vi "LoadWaveform.vi"() -> ()   [LabVIEW 2013]
panel:
  in  "Tab Control 2":enum32{"Main TEK", "load colored noise"}(tab)
  in  "channel 2":cluster{"output":bool}
  in  "channel 1":T1={"Modulation Waveform (1: Sine)"=200, "modulation"=FALSE, "output"=FALSE} {"Modulation Waveform (1: Sine)" items=["Sine"=1, "Square"=2, "Triangle"=3, "Ramp Up"=4, "Ramp Down"=5, "Noise"=100, "Arbitrary User1"=200, "Arbitrary User2"=201, "Arbitrary User3"=202, "Arbitrary User4"=203, "Edit Memory"=204]}
  in  "outpout mode":i32(ring) items=["Standard Waveform", "Arbitrary Waveform"]
  in  "configuration main":bool
  in  "amplitude (1)":dbl=1.0
  in  "dc offset (0.00)":dbl
  in  "frequency (1000000)":dbl=1000000.0
  in  "start phase (0.00)":dbl
  in  "amplitude (1) 2":dbl=1.0 caption="amplitude (1)"
  in  "dc offset (0.00) 2":dbl caption="dc offset (0.00)"
  in  "frequency (1000000) 2":dbl=1000000.0 caption="frequency (1000000)"
  in  "start phase (0.00) 2":dbl caption="start phase (0.00)"
  out "Noise density":dbl[](graph)
  in  "slot (0: Slot 1)":i32(ring) caption="USER (0: Slot 1)" items=["Slot 1", "Slot 2", "Slot 3", "Slot 4"]
  in  "gain (0.5)":dbl=0.5
  in  "offset (0.00)":dbl
  in  "sample rate (1000000000)":dbl=1000000000.0
  in  "loading on channel 1":bool
  in  "Waveform Size (1000)":i32=1000
  in  "waveform generation":bool
  out "min waveform size":i32
  out "max waveform size":i32
  out "waveform quantum":i32
  out "max number of waveforms":i32
  out "transfer error":errorcluster caption="error out" {"code" format="%.0x"}
  in  "resource name":refnum<k15>
  in  "Stop Button":bool
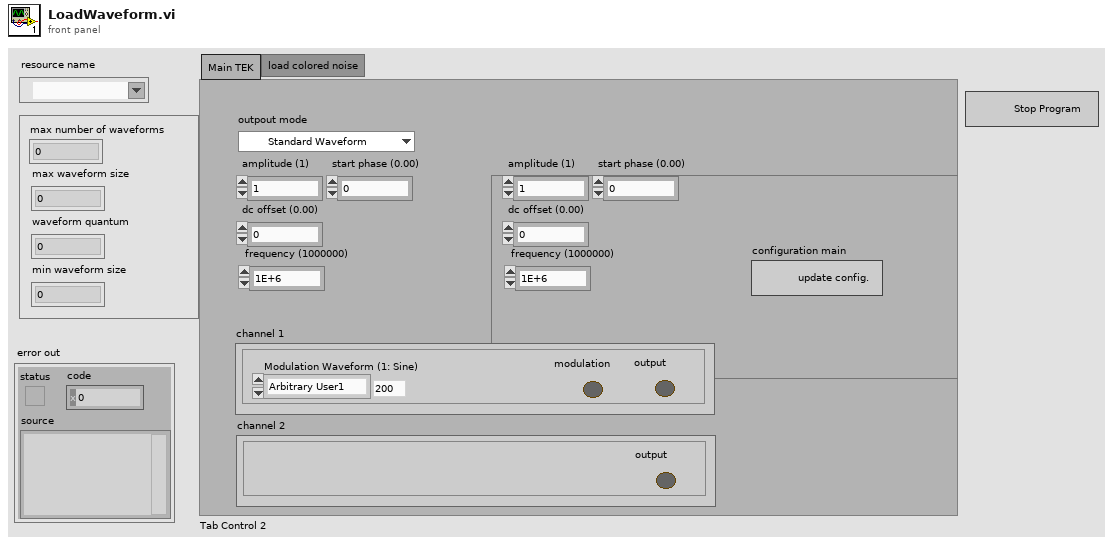
[diagram p1: front panel]
types:
  T1 = cluster{"Modulation Waveform (1: Sine)":i32, "modulation":bool, "output":bool}
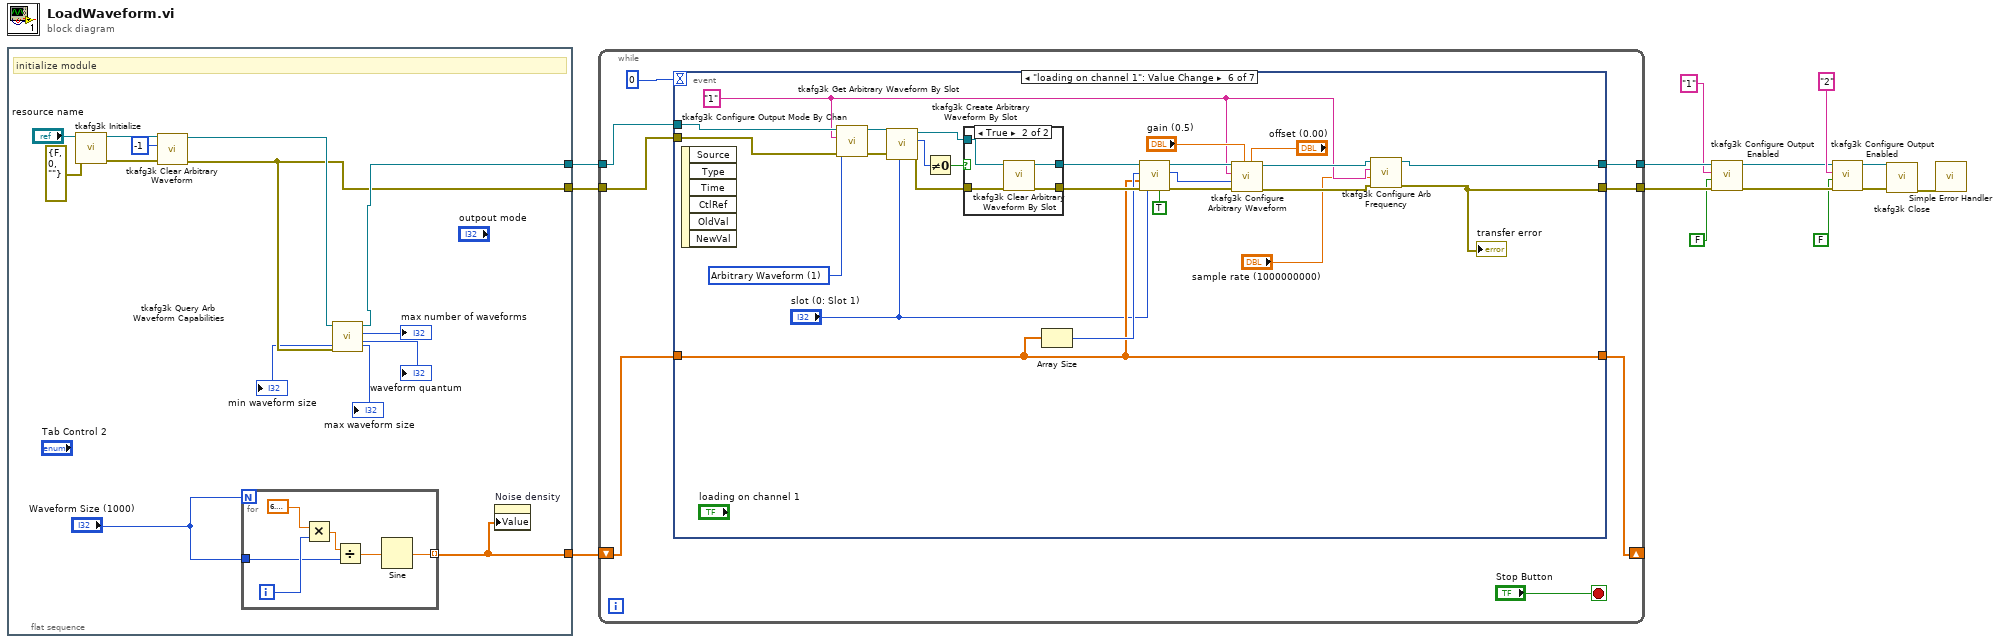
[diagram p0: block diagram]
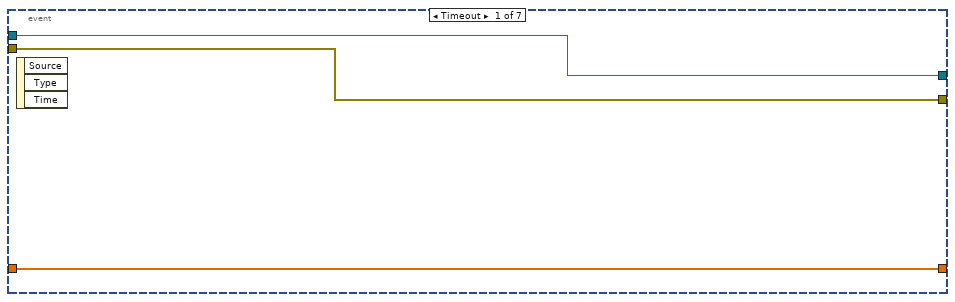
[diagram p2: hidden frame]
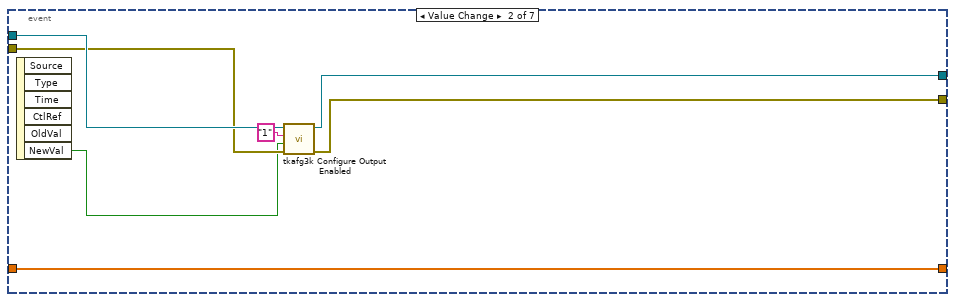
[diagram p3: hidden frame]
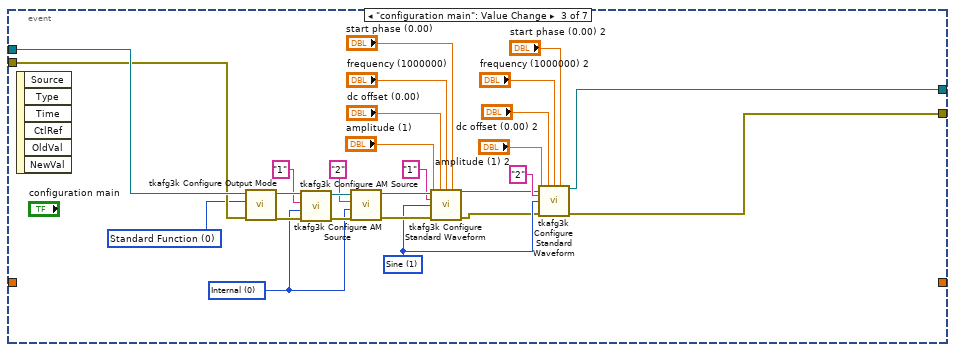
[diagram p4: hidden frame]
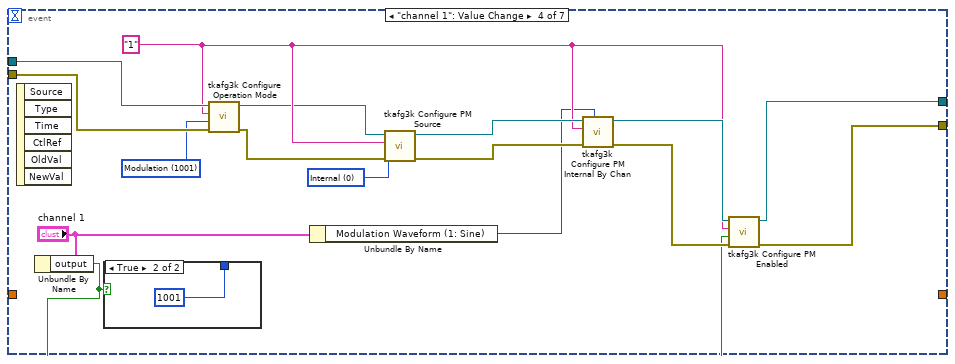
[diagram p5: hidden frame]
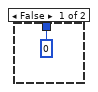
[diagram p6: hidden frame]
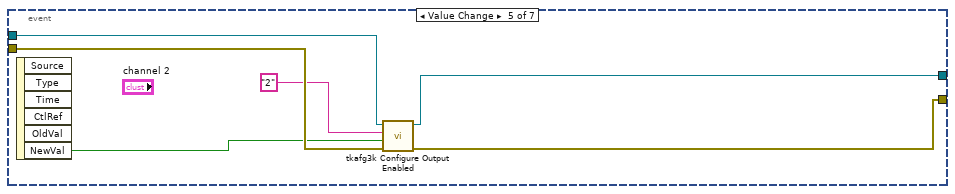
[diagram p7: hidden frame]
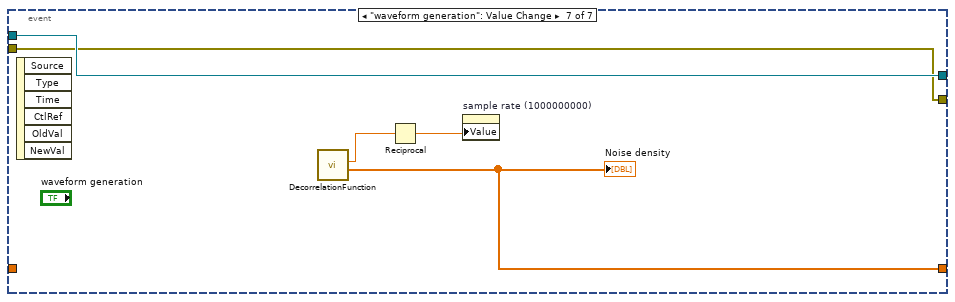
[diagram p9: hidden frame]
diagram:
  n1 = flat-sequence {
    tunnel: [w22] -> w10
    tunnel: [w21] -> w9
    tunnel: [w14] -> w5
    frame #0 {
      # "initialize module"
      n2 = call <instrlib>:"tkafg3k Initialize.vi"("error in (no error)"=errorcluster {"status"=FALSE, "code"=0, "source"=""}, "resource name"="resource name") -> ("error out"=w24:errorcluster, "instrument handle out"=w26:refnum<k15>)  [unwired: 8 in]
      n3 = call <instrlib>:"tkafg3k Clear Arbitrary Waveform.vi"("error in (no error)"=w24, "waveform handle"=-1, "instrument handle"=w26) -> ("error out"=w21:errorcluster, "instrument handle out"=w23:refnum<k15>)  [unwired: 7 in]
      n4 = for {
        N: "Waveform Size (1000)" -> [_]
        tunnel: "Waveform Size (1000)" -> [w29]
        tunnel: [w28] -> w14 mode=indexing
        i -> [w30]
        n5 = Multiply(x=6.283185307179586, y=w30) -> (x*y=w31:dbl)
        n6 = Divide(x=w31, y=w29) -> (x/y=w32:dbl)
        n7 = Sine(x=w32) -> (sin(x)=w28:dbl)
      }
      n8 = call <instrlib>:"tkafg3k Query Arb Waveform Capabilities.vi"("error in (no error)"=w21, "instrument handle"=w23) -> ("waveform quantum"=→"waveform quantum":i32, "max number of waveforms"=→"max number of waveforms":i32, "instrument handle out"=w22:refnum<k15>, "max waveform size"=→"max waveform size":i32, "min waveform size"=→"min waveform size":i32)  [unwired: 4 in, 1 out]
      n9 = property on="Noise density" class="WFGraph (strict)"("Value"=w14) -> ()  [unwired: 2 in, 2 out]
    }
  }
  n10 = while {
    tunnel: w10 -> [w40]
    tunnel: [w39] -> w4
    tunnel: w9 -> [w37]
    tunnel: [w36] -> w8
    shift-right: [w34] -> _
    shift-left: w5 -> [w35]
    stop <- "Stop Button" stop-if-true
    n11 = event shown="[5] \"loading on channel 1\": Value Change" {
      selector: _ -> [_ _ _ _ _ _ _]
      dyn-events: _ -> [_ _ _ _ _ _ _]
      timeout: 0 -> [_ _ _ _ _ _ _]
      tunnel: w40 -> [w43 w51 w78 w94 w102 w121 w139]
      tunnel: [w43 w50 w53 w84 w100 w104 w139] -> w39
      tunnel: w37 -> [w44 w48 w77 w93 w101 w120 w138]
      tunnel: [w44 w47 w52 w83 w99 w105 w138] -> w36
      tunnel: w35 -> [w42 w46 _ _ _ w116 _]
      tunnel: [w42 w46 _ _ _ w116 w137] -> w34
      event Timeout {
        n12 = event-data() -> ()  [unwired: 1 in, 3 out]
      }
      event "channel 1.output": Value Change {
        n13 = event-data() -> ("NewVal"=w45:bool)  [unwired: 1 in, 5 out]
        n14 = call <instrlib>:"tkafg3k Configure Output Enabled.vi"("error in (no error)"=w48, "channel enabled (True)"=w45, "channel name (\"1\")"="1" ("channel name (\"1\")"), "instrument handle"=w51) -> ("error out"=w47:errorcluster, "instrument handle out"=w50:refnum<k15>)  [unwired: 6 in]
      }
      event "configuration main": Value Change {
        w60 = 1 items=["Sine"=1, "Square"=2, "Pulse"=1002, "Ramp"=1001, "Noise"=1003, "DC"=6, "Sin(x)/x"=1004, "Gaussian"=1005, "Lorentz"=1006, "Exponential Rise"=1007, "Exponential Decay"=1008, "Haversine"=1009] ("waveform (1: Sine)")
        w69 = 0 items=["Internal", "External"] ("source (0: Internal)")
        w76 = 0 items=["Standard Function", "Arbitrary Waveform"] ("output mode (0: Standard Function)")
        n15 = event-data() -> ()  [unwired: 1 in, 6 out]
        n16 = call <instrlib>:"tkafg3k Configure Output Mode.vi"("error in (no error)"=w77, "output mode (0: Standard Function)"=w76, "instrument handle"=w78) -> ("error out"=w74:errorcluster, "instrument handle out"=w75:refnum<k15>)  [unwired: 7 in]
        n17 = call <instrlib>:"tkafg3k Configure AM Source.vi"("error in (no error)"=w74, "source (0: Internal)"=w69, "channel name (\"1\")"="1" ("channel name (\"1\")"), "instrument handle"=w75) -> ("error out"=w73:errorcluster, "instrument handle out"=w72:refnum<k15>)  [unwired: 6 in]
        n18 = call <instrlib>:"tkafg3k Configure AM Source.vi"("error in (no error)"=w73, "source (0: Internal)"=w69, "channel name (\"1\")"="2" ("channel name (\"1\")"), "instrument handle"=w72) -> ("error out"=w66:errorcluster, "instrument handle out"=w68:refnum<k15>)  [unwired: 6 in]
        n19 = call <instrlib>:"tkafg3k Configure Standard Waveform.vi"("instrument handle"=w68, "dc offset (0.00)"="dc offset (0.00)", "frequency (1000000)"="frequency (1000000)", "start phase (0.00)"="start phase (0.00)", "channel name (\"1\")"="1" ("channel name (\"1\")"), "waveform (1: Sine)"=w60, "amplitude (1)"="amplitude (1)", "error in (no error)"=w66) -> ("instrument handle out"=w58:refnum<k15>, "error out"=w59:errorcluster)  [unwired: 6 in]
        n20 = call <instrlib>:"tkafg3k Configure Standard Waveform.vi"("instrument handle"=w58, "dc offset (0.00)"="dc offset (0.00) 2", "frequency (1000000)"="frequency (1000000) 2", "start phase (0.00)"="start phase (0.00) 2", "channel name (\"1\")"="2" ("channel name (\"1\")"), "waveform (1: Sine)"=w60, "amplitude (1)"="amplitude (1) 2", "error in (no error)"=w59) -> ("instrument handle out"=w53:refnum<k15>, "error out"=w52:errorcluster)  [unwired: 6 in]
      }
      event "channel 1": Value Change {
        w79 = 1001 items=["Continuous"=0, "Modulation"=1001, "Sweep"=1002, "Burst"=1] ("operation mode (0: Continuous)")
        w92 = 0 items=["Internal", "External"] ("Source (0: Internal)")
        w86 = "1" ("channel name (\"1\")")
        n21 = event-data() -> ()  [unwired: 1 in, 6 out]
        n22 = Unbundle By Name("channel 1") -> ("output"=w82:bool)
        n23 = case shown="True" w82 {
          tunnel: [0 ("operation mode channel 3") 1001 ("operation mode channel 3")] -> _
          frame False {
          }
          frame True {
          }
        }
        n24 = call <instrlib>:"tkafg3k Configure Operation Mode.vi"("error in (no error)"=w93, "operation mode (0: Continuous)"=w79, "channel name (\"1\")"=w86, "instrument handle"=w94) -> ("error out"=w91:errorcluster, "instrument handle out"=w85:refnum<k15>)  [unwired: 6 in]
        n25 = Unbundle By Name("channel 1") -> ("Modulation Waveform (1: Sine)"=w81:i32)
        n26 = call <instrlib>:"tkafg3k Configure PM Source.vi"("error in (no error)"=w91, "Source (0: Internal)"=w92, "Channel Name (\"1\")"=w86, "instrument handle"=w85) -> ("error out"=w89:errorcluster, "instrument handle out"=w90:refnum<k15>)  [unwired: 6 in]
        n27 = call <instrlib>:"tkafg3k Configure PM Internal By Chan.vi"("Modulation Waveform (1: Sine)"=w81, "error in (no error)"=w89, "Channel Name (\"1\")"=w86, "instrument handle"=w90) -> ("error out"=w87:errorcluster, "instrument handle out"=w88:refnum<k15>)  [unwired: 6 in]
        n28 = call <instrlib>:"tkafg3k Configure PM Enabled.vi"("error in (no error)"=w87, "Enabled (True)"=w82, "Channel Name (\"1\")"=w86, "instrument handle"=w88) -> ("error out"=w83:errorcluster, "instrument handle out"=w84:refnum<k15>)  [unwired: 6 in]
      }
      event "channel 2.output": Value Change {
        n29 = event-data() -> ("NewVal"=w97:bool)  [unwired: 1 in, 5 out]
        n30 = call <instrlib>:"tkafg3k Configure Output Enabled.vi"("error in (no error)"=w101, "channel enabled (True)"=w97, "channel name (\"1\")"="2" ("channel name (\"1\")"), "instrument handle"=w102) -> ("error out"=w99:errorcluster, "instrument handle out"=w100:refnum<k15>)  [unwired: 6 in]
      }
      event "loading on channel 1": Value Change {
        w128 = 1 items=["Standard Function", "Arbitrary Waveform"] ("Output Mode (0: Standard Function)")
        w107 = "1" ("Channel Name (\"1\")")
        n31 = event-data() -> ()  [unwired: 1 in, 6 out]
        n32 = call <instrlib>:"tkafg3k Configure Output Mode By Chan.vi"("error in (no error)"=w120, "Output Mode (0: Standard Function)"=w128, "Channel Name (\"1\")"=w107, "instrument handle"=w121) -> ("error out"=w126:errorcluster, "instrument handle out"=w127:refnum<k15>)  [unwired: 6 in]
        n33 = call <instrlib>:"tkafg3k Get Arbitrary Waveform By Slot.vi"("slot (0: Slot 1)"="slot (0: Slot 1)", "error in (no error)"=w126, "instrument handle"=w127) -> ("error out"=w125:errorcluster, "waveform handle"=w122:i32, "instrument handle out"=w124:refnum<k15>)  [unwired: 6 in]
        n34 = Not Equal To 0?(x=w122) -> (x != 0?=w123:bool)
        n35 = case shown="True" w123 {
          tunnel: w124 -> [w130 w134]
          tunnel: w125 -> [w129 w133]
          tunnel: [w130 w132] -> w119
          tunnel: [w129 w131] -> w118
          frame False {
          }
          frame True {
            n36 = call <instrlib>:"tkafg3k Clear Arbitrary Waveform By Slot.vi"("error in (no error)"=w133, "instrument handle"=w134) -> ("error out"=w131:errorcluster, "instrument handle out"=w132:refnum<k15>)  [unwired: 8 in]
          }
        }
        n37 = Array Size(array=w116) -> (size(s)=w117:i32)
        n38 = call <instrlib>:"tkafg3k Create Arbitrary Waveform By Slot.vi"("overwrite (False)"=TRUE, "slot (0: Slot 1)"="slot (0: Slot 1)", "error in (no error)"=w118, "waveform data array"=w116, "waveform size (1000)"=w117, "instrument handle"=w119) -> ("error out"=w111:errorcluster, "waveform handle"=w112:i32, "instrument handle out"=w113:refnum<k15>)  [unwired: 3 in]
        n39 = call <instrlib>:"tkafg3k Configure Arbitrary Waveform.vi"("offset (0.00)"="offset (0.00)", "gain (0.5)"="gain (0.5)", "error in (no error)"=w111, "waveform handle"=w112, "channel name (\"1\")"=w107, "instrument handle"=w113) -> ("error out"=w106:errorcluster, "instrument handle out"=w108:refnum<k15>)  [unwired: 4 in]
        n40 = call <instrlib>:"tkafg3k Configure Arb Frequency.vi"("error in (no error)"=w106, "frequency (1000000)"="sample rate (1000000000)", "channel name (\"1\")"=w107, "instrument handle"=w108) -> ("error out"=w105:errorcluster, "instrument handle out"=w104:refnum<k15>)  [unwired: 6 in]
        "transfer error" <- w105
      }
      event "waveform generation": Value Change {
        n41 = event-data() -> ()  [unwired: 1 in, 6 out]
        n42 = call "DecorrelationFunction.vi"() -> ("waveform"=w137:dbl[], "temporal window (s)"=w136:dbl)  [unwired: 10 in]
        "Noise density" <- w137
        n43 = Reciprocal(x=w136) -> (1/x=w135:dbl)
        n44 = property on="sample rate (1000000000)" class="DigNum (strict)"("Value"=w135) -> ()  [unwired: 2 in, 2 out]
      }
    }
  }
  n45 = call <instrlib>:"tkafg3k Configure Output Enabled.vi"("channel enabled (True)"=FALSE, "channel name (\"1\")"="1" ("channel name (\"1\")"), "instrument handle"=w4) -> ("instrument handle out"=w3:refnum<k15>)  [unwired: 7 in, 1 out]
  n46 = call <instrlib>:"tkafg3k Configure Output Enabled.vi"("error in (no error)"=w8, "channel enabled (True)"=FALSE, "channel name (\"1\")"="2" ("channel name (\"1\")"), "instrument handle"=w3) -> ("error out"=w13:errorcluster, "instrument handle out"=w12:refnum<k15>)  [unwired: 6 in]
  n47 = call <instrlib>:"tkafg3k Close.vi"("error in (no error)"=w13, "instrument handle"=w12) -> ("error out"=w11:errorcluster)  [unwired: 9 in]
  n48 = call <vilib>:"Simple Error Handler.vi"("error in (no error)"=w11) -> ()  [unwired: 1 in, 8 out]
